vi "Enqueue Data.vi"(7 "is High Priority?":bool, 8 "error in (no error)":errorcluster, 9 "Data":variant, 10 "Message":string, 11 "queue in":refnum<queue>) -> (0 "error out":errorcluster, 3 "queue out":refnum<queue>)   [LabVIEW 2014, in "Queues Lib.lvlib"]
uses:
  Queues Lib.lvlib
  Queues Message Type Def.ctl
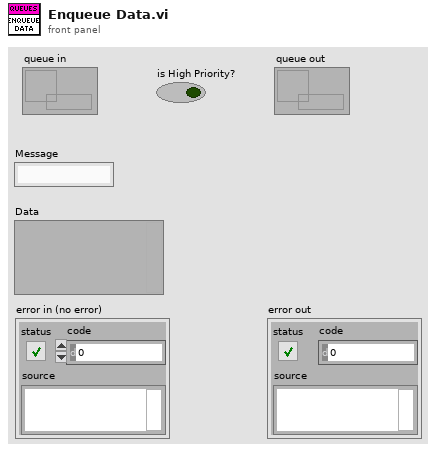
[diagram p1: front panel]
types:
  T1 = typedef "Queues Lib.lvlib/Queues Message Type Def.ctl" = cluster{"Message":string, "Data":variant}
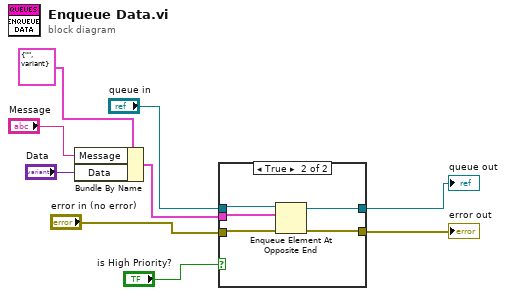
[diagram p0: block diagram]
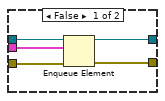
[diagram p2: hidden frame]
diagram:
  n1 = Bundle By Name(cluster=T1 {"Message"="", "Data"=variant} ("Queue Message"), "Message"="Message", "Data"="Data") -> (w2:T1)
  n2 = case shown="True" "is High Priority?" {
    tunnel: [w14 w16] -> w7
    tunnel: "error in (no error)" -> [w13 w17]
    tunnel: [w12 w15] -> w5
    tunnel: "queue in" -> [w11 w19]
    tunnel: w2 -> [w10 w18]
    frame False {
      n3 = Enqueue Element(queue=w11, element=w10, error in (no error)=w13) -> (queue out=w12:refnum<queue>, error out=w14:errorcluster)  [unwired: 1 in, 1 out]
    }
    frame True {
      n4 = Enqueue Element At Opposite End(queue=w19, element=w18, error in (no error)=w17) -> (queue out=w15:refnum<queue>, error out=w16:errorcluster)  [unwired: 1 in, 1 out]
    }
  }
  "error out" <- w7
  "queue out" <- w5
